vi "LaunchAIServer.vi"(8 "error in (no error)":errorcluster, 11 "InferenceTCP in":refnum<class "InferenceTCP.lvclass">) -> (0 "error out":errorcluster, 3 "InferenceTCP out":refnum<class "InferenceTCP.lvclass">)   [LabVIEW 2019, in "InferenceTCP.lvlib" / "InferenceTCP.lvclass"]
uses:
  InferenceTCP.lvclass
  InferenceTCP.lvclass/InferenceTCP.ctl
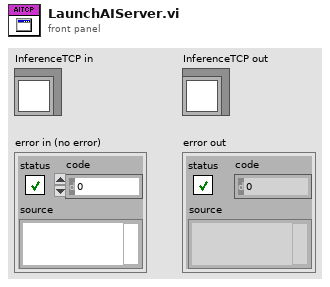
[diagram p1: front panel]
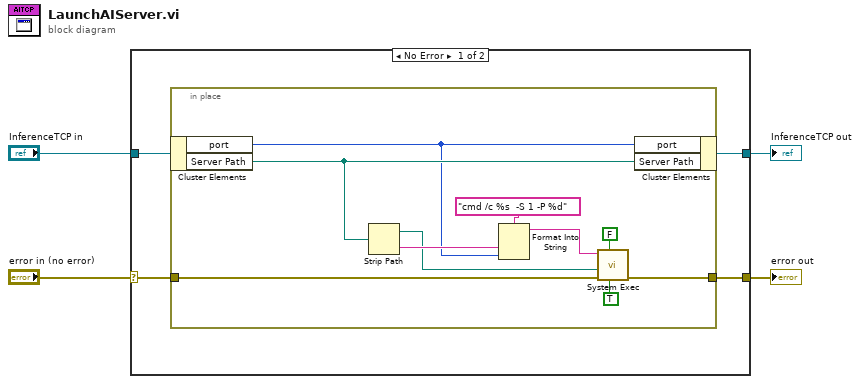
[diagram p0: block diagram]
diagram:
  n1 = case shown="No Error" "error in (no error)" {
    selector: "error in (no error)" -> [w6 w20]
    tunnel: [w5 w20] -> w3
    tunnel: [w7 w19] -> w1
    tunnel: "InferenceTCP in" -> [w8 w19]
    frame No Error {
      n2 = in-place {
        in-place-border: w6 -> [w10]
        in-place-border: [w9] -> w5
        n3 = in-place-cluster #1(w8) -> ("port"=w11:u16, "Server Path"=w16:path)
        n4 = Strip Path(path=w16) -> (stripped path=w13:path, name=w14:string)
        n5 = Format Into String(format string="cmd /c %s  -S 1 -P %d" ("command line"), w14, w11) -> (resulting string=w12:string)  [unwired: 2 in, 1 out]
        n6 = call <vilib>:"System Exec.vi"("run minimized? (F)"=TRUE, "wait until completion? (T)"=FALSE, "error in (no error)"=w10, "working directory"=w13, "command line"=w12) -> ("error out"=w9:errorcluster)  [unwired: 3 in, 3 out]
        n7 = in-place-cluster #1("port"=w11, "Server Path"=w16) -> (w7:refnum<class "InferenceTCP.lvclass">)
      }
    }
    frame Error {
    }
  }
  "error out" <- w3
  "InferenceTCP out" <- w1
